vi "Delete Oldest File.vi"(8 "error in":errorcluster, 10 "pattern":string, 11 "path":path) -> (0 "error out":errorcluster, 3 "path out":path)   [LabVIEW 2023]
doc: "Removes oldest *FILE* in a directory ignoring Mac files .DS_Store, .Icon and .localized. Should not need to use unix system calls and is in pure G! Can be restricted to specific pattern files.\nScott Hannahs <sth@magnet.fsu.edu>"
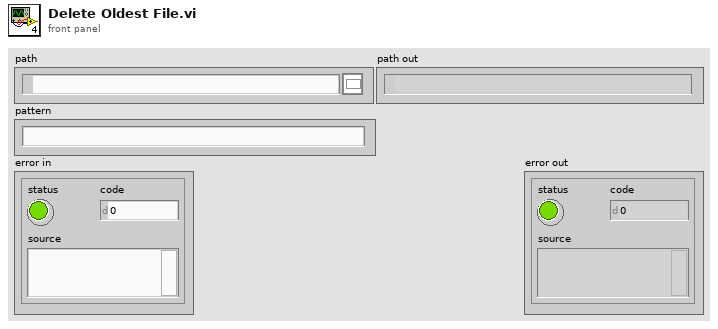
[diagram p1: front panel]
types:
  T1 = cluster{"last mod":timestamp, "appended path":path}
  T2 = cluster{"last mod":timestamp, "appended path":path}[]
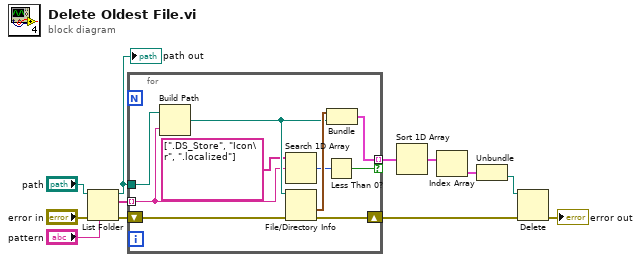
[diagram p0: block diagram]
diagram:
  n1 = List Folder(path="path", pattern="pattern", error in="error in") -> (path out=w1:path, filenames=w12:string[], error out=w3:errorcluster)  [unwired: 1 in, 1 out]
  "path out" <- w1
  n2 = for {
    tunnel: w12 -> [w18] mode=indexing
    tunnel: w1 -> [w22]
    tunnel: [w19] -> w10 mode=indexing if=w15
    shift-right: [w13] -> w2
    shift-left: w3 -> [w14]
    n3 = Build Path(base path=w22, name or relative path=w18) -> (appended path=w20:path)
    n4 = Search 1D Array(1D array=string[] [".DS_Store", "Icon\r", ".localized"], element=w18) -> (index of element=w16:i32)  [unwired: 1 in]
    n5 = File/Directory Info(path=w20, error in=w14) -> (last mod=w21:timestamp, error out=w13:errorcluster)  [unwired: 5 out]
    n6 = Less Than 0?(x=w16) -> (x < 0?=w15:bool)
    n7 = Bundle("last mod"=w21, "appended path"=w20) -> (w19:T1)  [unwired: 1 in]
  }
  n8 = Sort 1D Array(array=w10) -> (sorted array=w9:T2)
  n9 = Index Array(array=w9) -> (element=w8:T1)  [unwired: 1 in]
  n10 = Unbundle(w8) -> ("appended path"=w7:path)  [unwired: 1 out]
  n11 = Delete(path (use dialog)=w7, error in=w2) -> (error out=→"error out":errorcluster)  [unwired: 3 in, 2 out]
